vi "_Get Image.vi"(6 "Image Type (U16)":T1=7 items=["Grayscale (U8)", "Grayscale (I16)", "Grayscale (SGL)", "Complex (CSG)", "RGB (U32)", "HSL (U32)", "RGB (U64)", "Grayscale (U16)"], 7 "XY Resolution":i32, 8 "error in":errorcluster, 9 "Image File":path, 10 "Image Name":string, 11 "Image":T3) -> (0 "error out":errorcluster, 1 "Image Pixels (Float)":dbl[][](array[numeric]) format="%.2f", 2 "Image Pixels (U16)":u16[][](array[numeric]), 3 "Image Out":T2)   [LabVIEW 2023]
uses:
  _Images.ctl
  <vilib>/vision/Image Controls.llb/IMAQ Image.ctl
  <vilib>/vision/NI_Vision_Development_Module.lvlib
panel:
  out "Image":T2(plugin-control)
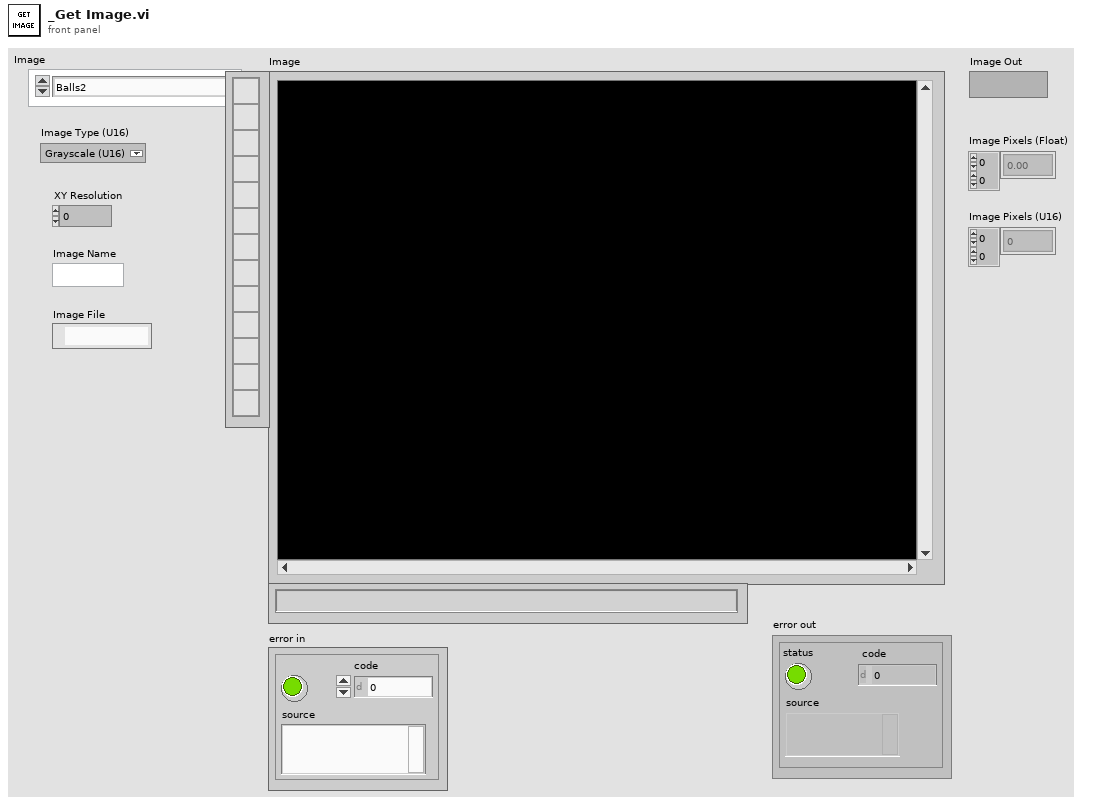
[diagram p1: front panel]
types:
  T1 = typedef "Image Type" = u32
  T2 = typedef "IMAQ Image.ctl" = refnum<image>
  T3 = typedef "_Images.ctl" = enum16{"Balls2", "Battery1", "Battery2", "Connector1", "Subwoofer1", "Subwoofer2", "Subwoofer3", "Subwoofer4", "Hase1", "Lamp1", "Lamp2", "Mouse1", "PhotoLens1", "Po1", "PowerSupply1", "Router", "--- Step Wedges ---", "Stepwedge1", "Stepwedge2", "Stepwedge3", "--- Fusion ---", "Fusion160kV", "Fusion2-120kV", "Fusion2-320kV", "Fusion300kV", "FusionPart1-120kV", "FusionPart1-180kV", "--- PART 01 ---", "Part1", "Part2", "Part3", "Part4", "Part5", "Part6", "Part7", "Part8", "--- Different Integrations ---", "Step2737-02Int", "Step2737-04Int", "Step2737-08Int", "Step2737-16Int", "Step2737-32Int", "Step2737-64Int"}
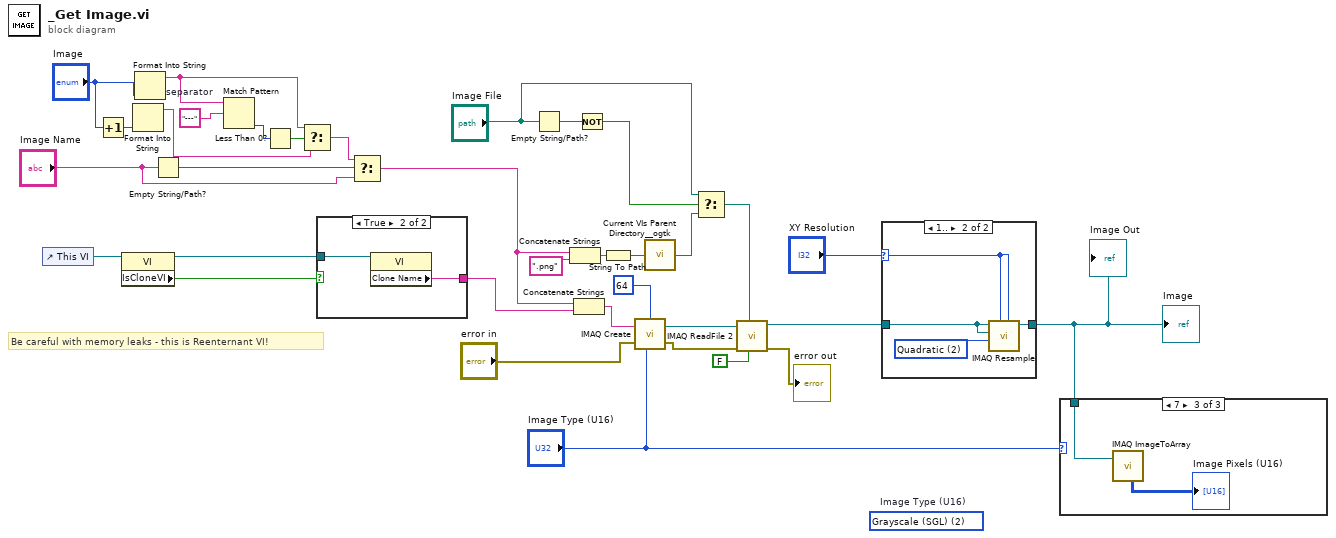
[diagram p0: block diagram]
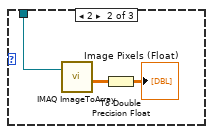
[diagram p3: hidden frame]
diagram:
  w8 = "---"  # separator
  (unwired) T1 2 items=["Grayscale (U8)", "Grayscale (I16)", "Grayscale (SGL)", "Complex (CSG)", "RGB (U32)", "HSL (U32)", "RGB (U64)", "Grayscale (U16)"]  # Image Type (U16)
  # "Be careful with memory leaks - this is Reenternant VI!"
  n1 = control-ref of="This VI"() -> (w24:refnum<vi>)
  n2 = Increment(x="Image") -> (x+1=w3:T3)
  n3 = property class="VI"(reference=w24) -> (reference out=w23:refnum<vi>, "IsCloneVI"=w22:bool)  [unwired: 1 in, 1 out]
  n4 = Format Into String(w3) -> (resulting string=w2:string)  [unwired: 3 in, 1 out]
  n5 = Format Into String("Image") -> (resulting string=w5:string)  [unwired: 3 in, 1 out]
  n6 = Empty String/Path?(string/path="Image Name") -> (empty?=w17:bool)
  n7 = Match Pattern(string=w5, regular expression=w8) -> (offset past match=w7:i32)  [unwired: 1 in, 3 out]
  n8 = Less Than 0?(x=w7) -> (x < 0?=w6:bool)
  n9 = Select(t=w5, s=w6, f=w2) -> (s? t:f=w1:string)
  n10 = case shown="True" w22 {
    tunnel: [_ w36] -> w21
    tunnel: w23 -> [_ w35]
    frame False {
    }
    frame True {
      n11 = property class="VI"(reference=w35) -> ("Clone Name"=w36:string)  [unwired: 1 in, 2 out]
    }
  }
  n12 = Select(t=w1, s=w17, f="Image Name") -> (s? t:f=w19:string)
  n13 = Empty String/Path?(string/path="Image File") -> (empty?=w13:bool)
  n14 = Concatenate Strings(w19, ".png" ("string")) -> (w32:string)
  n15 = Concatenate Strings(w19, w21) -> (w20:string)
  n16 = Not(x=w13) -> (.not. x?=w11:bool)
  n17 = String To Path(string=w32) -> (path=w31:path)
  n18 = call "IMAQ Create"("Border Size"=64, "Image Name"=w20, "Image Type"="Image Type (U16)", "error in (no error)"="error in") -> ("New Image"=w34:T2, "error out"=w30:errorcluster)  [unwired: 1 in]
  n19 = call <userlib>:"Current VIs Parent Directory__ogtk.vi"("Relative path (.)"=w31) -> ("Parent Directory (+ Relative)"=w9:path)  [unwired: 4 in]
  n20 = Select(t="Image File", s=w11, f=w9) -> (s? t:f=w12:path)
  n21 = call "IMAQ ReadFile 2"("Use File Path Image Type"=FALSE, "File Path"=w12, "error in (no error)"=w30, "Image"=w34) -> ("error out"=→"error out":errorcluster, "Image Out"=w26:T2)  [unwired: 3 in, 3 out]
  n22 = case shown="1.." "XY Resolution" {
    selector: "XY Resolution" -> [_ w38]
    tunnel: [w37 w41] -> w14
    tunnel: w26 -> [w37 w40]
    frame ..0, Default {
    }
    frame 1.. {
      w39 = u32 2 items=["Zero Order", "Bi-Linear", "Quadratic", "Cubic Spline"] ("Interpolation Type")
      n23 = call "IMAQ Resample"("X Resolution"=w38, "Y Resolution"=w38, "Interpolation Type"=w39, "Image Dst"=w40, "Image Src"=w40) -> ("Image Dst Out"=w41:T2)  [unwired: 5 in, 1 out]
    }
  }
  "Image" <- w14
  "Image Out" <- w14
  n24 = case shown="7" "Image Type (U16)" {
    tunnel: w14 -> [_ w44 w46]
    frame 0, Default {
    }
    frame 2 {
      n25 = call "IMAQ ImageToArray"("Image"=w44) -> ("Image Pixels (Float)"=w43:sgl[][])  [unwired: 3 in, 4 out]
      n26 = To Double Precision Float(number=w43) -> (double precision float=→"Image Pixels (Float)":dbl[][])
    }
    frame 7 {
      n27 = call "IMAQ ImageToArray"("Image"=w46) -> ("Image Pixels (U16)"=→"Image Pixels (U16)":u16[][])  [unwired: 3 in, 4 out]
    }
  }
